vi "Signals.Scale.Raw.vi"(5 "Lookup":variant, 6 "Type":T1, 7 "Writes Ref":T2, 8 "error in":errorcluster, 11 "ID":u32) -> (0 "error out":errorcluster, 2 "Data":u8[](array[numeric]))   [LabVIEW 2019, in "Diagnostics Addon Engine.lvlib"]
uses:
  Diagnostics Addon Engine.lvlib
  <vilib>/NI/NIVS Inline Async API/_Data Access Engine/Data Access Engine/Types/Read.DVR.ctl
  <vilib>/NI/NIVS Inline Async API/_Data Access Engine/Access Type Classes/Read/Read.lvclass
  Addon Shared/Types/Type.ctl
  Addon Shared/Types/Frame.Lookup.Info.ctl
  <vilib>/NI/NIVS Inline Async API/_Data Access Engine/Access Type Classes/Read/Read.lvclass/Read.ctl
  <vilib>/NI/NIVS Inline Async API/_Data Access Engine/Data Access Engine/Methods/Read.Data.vi
  <vilib>/NI/NIVS Inline Async API/_Data Access Engine/Access Type Classes/Read/Read.ProcessData.vi
  Addon Shared/SubVIs/Constants.vi
  <vilib>/xnet/xnet.llb/XNET Convert (Signal to Frame CAN).vi
  Addon Shared/Diagnostics Addon Shared.lvlib
  <vilib>/NI/NIVS Inline Async API/_Data Access Engine/Data Access Engine/Data Access Engine.lvclass
  <vilib>/Utility/SystemLogging/NI_SystemLogging.lvlib
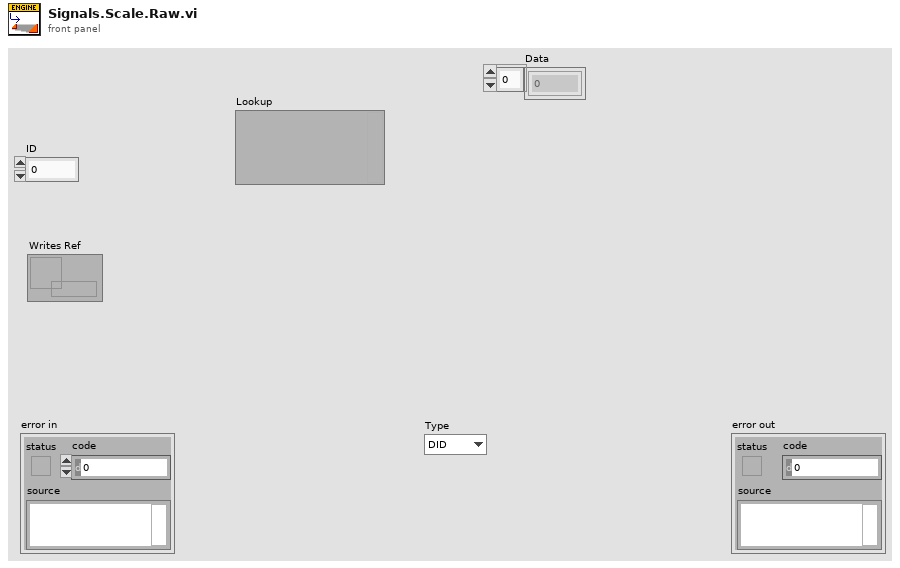
[diagram p1: front panel]
types:
  T1 = typedef "Diagnostics Addon Shared.lvlib/Type.ctl" = enum16{"DID", "CDID", "PID", "CPID", "Read Memory", "Write Memory", "IO Control", "Routine Start", "Routine Request", "Routine Stop", "User Defined", "DTC Control", "Clear DTCs", "Read DTCs", "Start DTCs", "DTC Change Count", "Tester Present", "Unlock ECU", "Reset ECU", "Diag Session Control", "Communication Control", "DPID Control", "Poll Control", "Diag CAN Control"}
  T2 = typedef "Data Access Engine.lvlib/Data Access Engine.lvclass/Read.DVR.ctl" = refnum<data-value>
  T3 = enum16{"Output/Write", "Input/Read", "Input/ReadWrite"}
  T4 = typedef "Diagnostics Addon Shared.lvlib/Frame.Lookup.Info.ctl" = cluster{"Offset":i32, "Length":i32, "ByteLength":u16}
  T5 = typedef "XNET Frame CAN.ctl" = cluster{"timestamp":timestamp, "payload":u8[], "identifier":u32, "type":T6, "extended?":bool, "echo?":bool}
  T6 = typedef "XNET Frame Type CAN.ctl" = u8
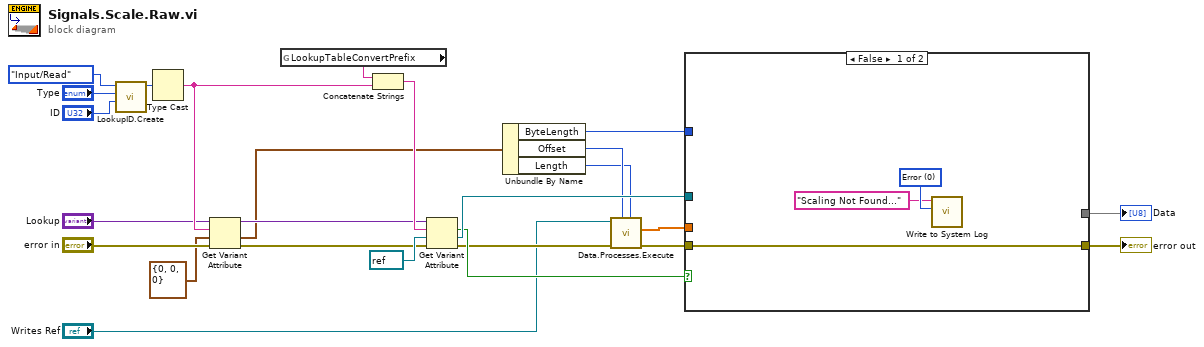
[diagram p0: block diagram]
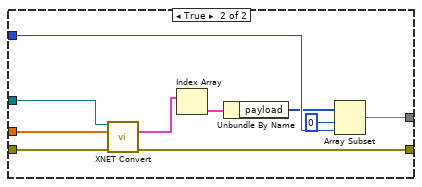
[diagram p2: hidden frame]
diagram:
  n1 = call "LookupID.Create.vi"("Serivce ID"="ID", "Service Type"="Type", "Direction"=T3."Input/Read") -> ("Result"=w2:u64)  [unwired: 8 in]
  n2 = Type Cast(x=w2) -> (*(type *) &x=w19:string)  [unwired: 1 in]
  n3 = Get Variant Attribute(Variant="Lookup", name=w19, default value (empty Variant)=T4 {"Offset"=0, "Length"=0, "ByteLength"=0} ("cluster"), error in="error in") -> (duplicate Variant=w18:variant, value=w13:T4, error out=w20:errorcluster)  [unwired: 1 out]
  n4 = global read "Constants.vi" "LookupTableConvertPrefix"() -> (w21:string)
  n5 = Concatenate Strings(w21, w19) -> (w22:string)
  n6 = Get Variant Attribute(Variant=w18, name=w22, default value (empty Variant)=refnum<k21> refnum ("DID Conversion"), error in=w20) -> (found=w11:bool, value=w14:refnum<k21>, error out=w7:errorcluster)  [unwired: 1 out]
  n7 = Unbundle By Name(w13) -> ("ByteLength"=w16:u16, "Offset"=w10:i32, "Length"=w9:i32)
  n8 = call-poly <vilib>:"Data.Processes.Execute.vi"("length"=w9, "index"=w10, "error in (no error)"=w7, "Ref"="Writes Ref") -> ("error out"=w6:errorcluster, "Values"=w8:dbl[])  [unwired: 5 in, 1 out]
  n9 = case shown="False" w11 {
    tunnel: w6 -> [w28 w38]
    tunnel: [w28 w32] -> w12
    tunnel: w8 -> [_ w34]
    tunnel: w14 -> [_ w37]
    tunnel: w16 -> [_ w35]
    tunnel: [_ w33] -> w15
    frame False {
      w27 = 0 items=["Error", "Warning", "Informational"] ("severity")
      n10 = call <vilib>:"Write to System Log.vi"("severity"=w27, "message"="Scaling Not Found..." ("Message")) -> ()  [unwired: 9 in, 1 out]
    }
    frame True {
      n11 = call-poly <vilib>:"XNET Convert.vi"("session in"=w37, "signal data"=w34, "error in (no error)"=w38) -> ("frame data"=w31:T5[], "error out"=w32:errorcluster)  [unwired: 9 in, 2 out]
      n12 = Index Array(array=w31) -> (element=w30:T5)  [unwired: 1 in]
      n13 = Unbundle By Name(w30) -> ("payload"=w29:u8[])
      n14 = Array Subset(array=w29, index=0, length=w35) -> (w33:u8[])
    }
  }
  "error out" <- w12
  "Data" <- w15
